vi "BatterySim_Execute.vi"(9 "Battery Resistance Ohms":dbl=0.03 format="%#_13g", 10 "Nominal Battery Voltage":dbl=12.0, 11 "Current":dbl) -> (3 "Voltage":dbl)   [LabVIEW 2019, in "Trajectory_Library.lvlib"]
doc: "LabVIEW single call function to simulate loaded battery voltage. \n\nInputs:\n - current -- double -- sum of all currents connected to this battery (amps)\n - nominalVoltage -- double -- The nominal battery voltage. (Volts) Usually 12v. (Default: 12)\n - Battery Resistance -- double -- The forward resistance of the battery. Most batteries are at or below 20 milliohms. (Ohms) (Default: 0.03)\n\nOutputs:\n - Voltage -- The battery's voltage under load."
uses:
  Trajectory_Library.lvlib
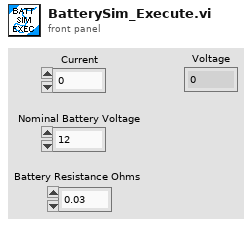
[diagram p1: front panel]
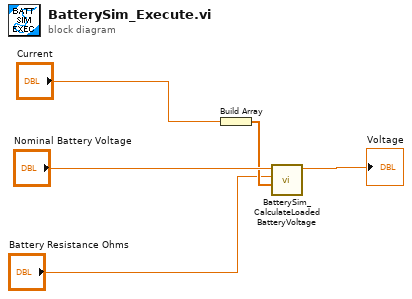
[diagram p0: block diagram]
diagram:
  n1 = Build Array("Current") -> (w2:dbl[])
  n2 = call "BatterySim_CalculateLoadedBatteryVoltage.vi"("Currents"=w2, "Resistance_Ohms"="Battery Resistance Ohms", "NominalVoltage"="Nominal Battery Voltage") -> ("Voltage"=→"Voltage":dbl)  [unwired: 8 in]
